vi "controller_FGV.vi"(5 "error in":errorcluster, 7 "PS3 Controls":T2 {"Left Analogue Stick X" scale=-32768.0..32768.0; "Left Analogue Stick Y" scale=32768.0..-32768.0; "Right Analogue Stick X" scale=-32768.0..32768.0; "Right Analogue Stick Y" scale=32768.0..-32768.0; "X Rotation" scale=-32768.0..32768.0; "Y Rotation" scale=-32768.0..32768.0; "L2 Pressure" scale=0.0..32768.0; "Numeric" format="%d°"}, 13 "Action":T1) -> (6 "Left Analogue Stick X":i32, 8 "Left Analogue Stick Y":i32, 10 "Right Analogue Stick Y":i32, 12 "Right Analogue Stick X":i32, 14 "Triangle":bool, 15 "Square":bool, 16 "X":bool, 17 "Circle":bool, 19 "error out":errorcluster)   [LabVIEW 2024]
uses:
  PS3 Controls.ctl
  backups BRIGHTLAB/CARNEVALI test3/Project_Brightlab_maschiatori/SLCMotors/FGV/FGV Actions.ctl
panel:
  out "PS Button":bool
  out "Start":bool
  out "Select":bool
  out "R3":bool
  out "L3":bool
  out "R2":bool
  out "L2":bool
  out "R1":bool
  out "L1":bool
  out "R2 Pressure":i32
  out "L2 Pressure":i32
  out "X Rotation":i32
  out "Y Rotation":i32
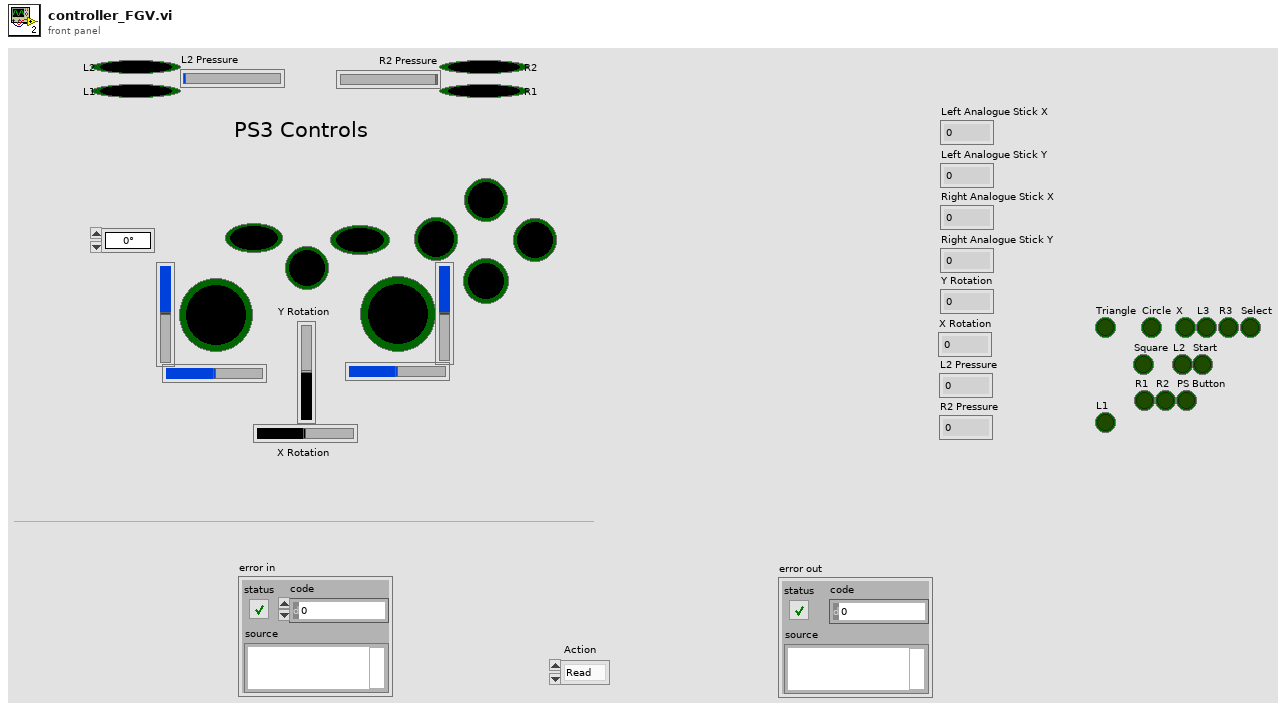
[diagram p1: front panel]
types:
  T1 = typedef "FGV Actions.ctl" = enum16{"Read", "Write"}
  T2 = typedef "PS3 Controls.ctl" = cluster{"Left Analogue Stick X":i32, "Left Analogue Stick Y":i32, "Right Analogue Stick X":i32, "Right Analogue Stick Y":i32, "Y Rotation":i32, "X Rotation":i32, "L2 Pressure":i32, "R2 Pressure":i32, "Triangle":bool, "Circle":bool, "X":bool, "Square":bool, "L1":bool, "R1":bool, "L2":bool, "R2":bool, "L3":bool, "R3":bool, "Select":bool, "Start":bool, "PS Button":bool, "Numeric":i32}
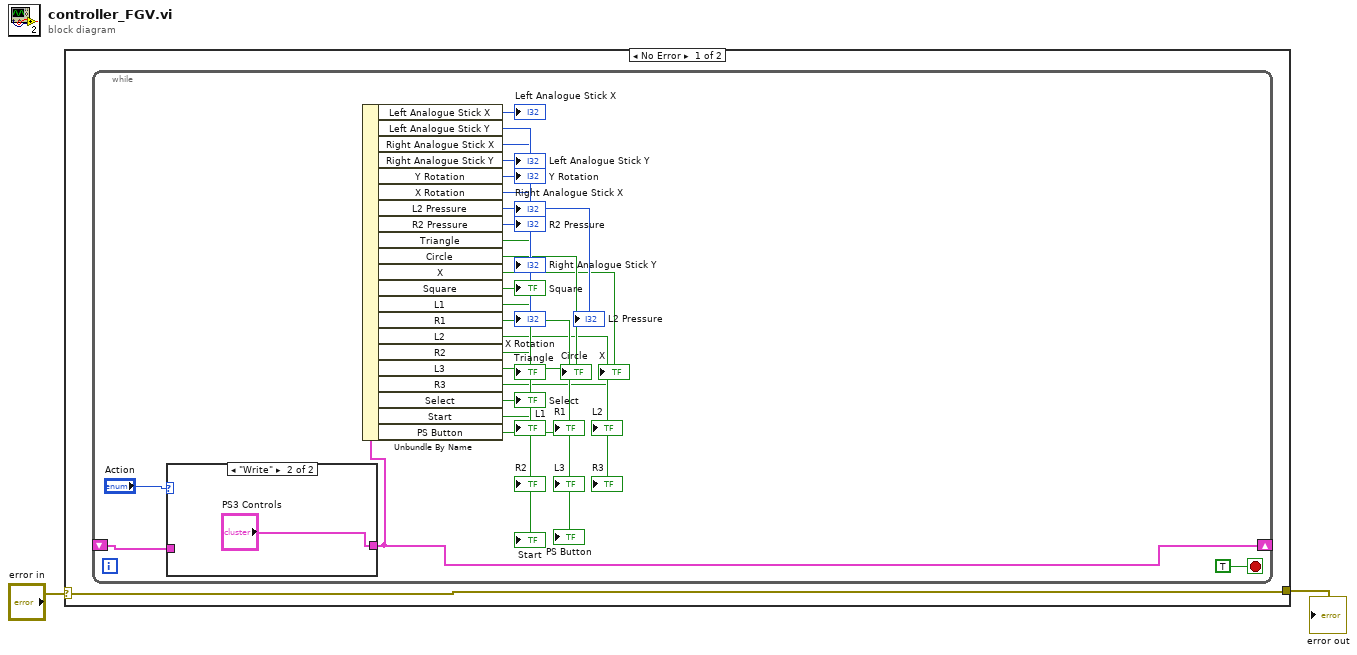
[diagram p0: block diagram]
diagram:
  n1 = case shown="No Error" "error in" {
    selector: "error in" -> [w3 w31]
    tunnel: [w3 w31] -> w1
    frame No Error {
      n2 = while {
        shift-right: [w5] -> _
        shift-left: _ -> [w27]
        stop <- TRUE stop-if-true
        n3 = case shown="\"Write\"" "Action" {
          tunnel: [w29 "PS3 Controls"] -> w5
          tunnel: w27 -> [w29 _]
          frame "Read", Default {
          }
          frame "Write" {
          }
        }
        n4 = Unbundle By Name(w5) -> ("Left Analogue Stick X"=→"Left Analogue Stick X":i32, "Left Analogue Stick Y"=→"Left Analogue Stick Y":i32, "Right Analogue Stick X"=→"Right Analogue Stick X":i32, "Right Analogue Stick Y"=→"Right Analogue Stick Y":i32, "Y Rotation"=→"Y Rotation":i32, "X Rotation"=→"X Rotation":i32, "L2 Pressure"=→"L2 Pressure":i32, "R2 Pressure"=→"R2 Pressure":i32, "Triangle"=→"Triangle":bool, "Circle"=→"Circle":bool, "X"=→"X":bool, "Square"=→"Square":bool, "L1"=→"L1":bool, "R1"=→"R1":bool, "L2"=→"L2":bool, "R2"=→"R2":bool, "L3"=→"L3":bool, "R3"=→"R3":bool, "Select"=→"Select":bool, "Start"=→"Start":bool, "PS Button"=→"PS Button":bool)
      }
    }
    frame Error {
    }
  }
  "error out" <- w1
